vi "sub_提取奇偶行2.vi"(0 "数组":dbl[][](array[numeric])=[[1.0, 2.0, 3.0, 4.0], [5.0, 6.0, 7.0, 8.0], [9.0, 10.0, 11.0, 12.0], [13.0, 14.0, 15.0, 16.0]]) -> (5 "奇数行一维数组":dbl[](array[numeric]) format="%.2f", 6 "偶数行一维数组":dbl[](array[numeric]) format="%.2f")   [LabVIEW 2015]
panel:
  out "偶数行":dbl[][](array[numeric])=[[5.0, 6.0, 7.0, 8.0], [13.0, 14.0, 15.0, 16.0]] format="%.2f"
  out "奇数行":dbl[][](array[numeric])=[[1.0, 2.0, 3.0, 4.0], [9.0, 10.0, 11.0, 12.0]] format="%.2f"
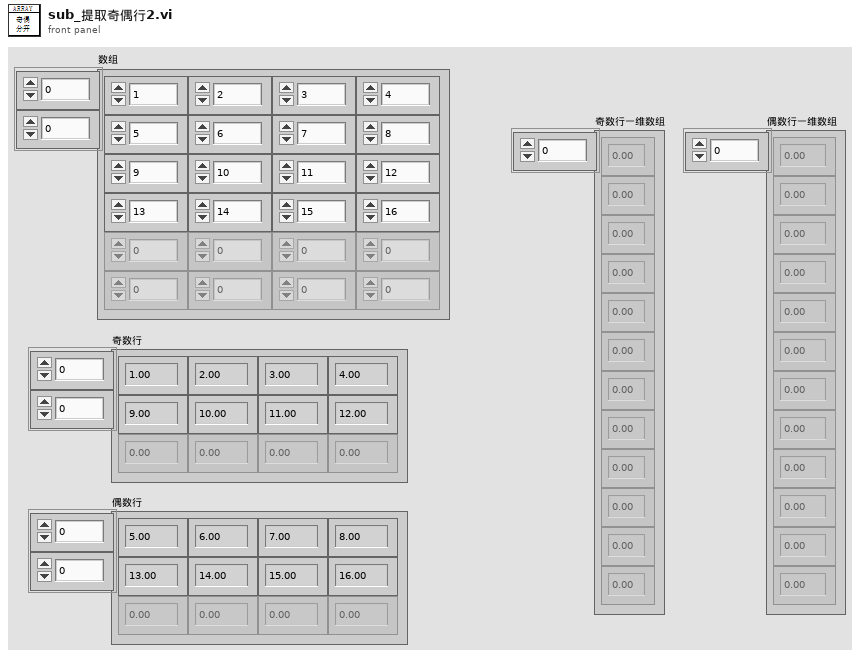
[diagram p1: front panel]
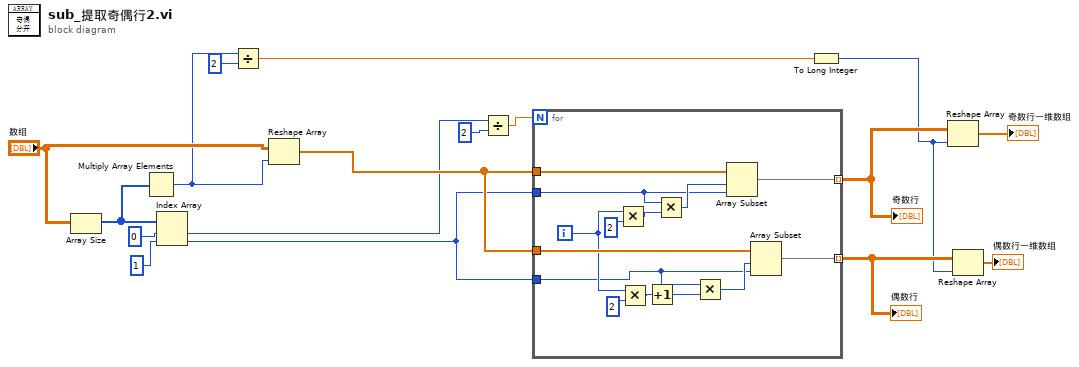
[diagram p0: block diagram]
diagram:
  n1 = Array Size(array="数组") -> (size(s)=w12:i32[])
  n2 = Multiply Array Elements(1:w12) -> (0:w10:i32)
  n3 = Index Array(array=w12, index #1=0 ("索引"), index #2=1 ("索引")) -> (element #1=w14:i32, element #2=w1:i32)
  n4 = Divide(x=w10, y=2) -> (x/y=w5:dbl)
  n5 = Reshape Array("数组", w10) -> (w15:dbl[])
  n6 = Divide(x=w14, y=2) -> (x/y=w4:dbl)
  n7 = for {
    N: w4 -> [_]
    tunnel: w15 -> [w31]
    tunnel: [w29] -> w11 mode=indexing
    tunnel: w15 -> [w24]
    tunnel: [w23] -> w8 mode=indexing
    tunnel: w1 -> [w18]
    tunnel: w1 -> [w19]
    i -> [w22]
    n8 = Multiply(x=w22, y=2) -> (x*y=w28:i32)
    n9 = Multiply(x=w22, y=2) -> (x*y=w25:i32)
    n10 = Increment(x=w25) -> (x+1=w20:i32)
    n11 = Multiply(x=w18, y=w28) -> (x*y=w30:i32)
    n12 = Multiply(x=w19, y=w20) -> (x*y=w21:i32)
    n13 = Array Subset(array=w31, index=w30, length=w18) -> (w29:dbl[])
    n14 = Array Subset(array=w24, index=w21, length=w19) -> (w23:dbl[])
  }
  "奇数行" <- w11
  "偶数行" <- w8
  n15 = To Long Integer(number=w5) -> (32bit integer=w3:i32)
  n16 = Reshape Array(w11, w3) -> (→"奇数行一维数组":dbl[])
  n17 = Reshape Array(w8, w3) -> (→"偶数行一维数组":dbl[])
